vi "Retrieve Category SubPanel Information.vi"(8 "error in (no error)":errorcluster, 10 "ListBox Selection":i32, 11 "Configuration in":refnum<class "Configuration.lvclass">) -> (0 "error out":errorcluster, 1 "Help Text":string, 2 "VI Refnum":refnum<vi>, 3 "Configuration Out":refnum<class "Configuration.lvclass">)   [LabVIEW 2016, in "Configuration.lvlib" / "Configuration.lvclass"]
uses:
  <userlib>/Configuration Dialog Actor/Configuration.lvclass
  <userlib>/Configuration Dialog Actor/Configuration.lvclass/Configuration.ctl
  <userlib>/Configuration Dialog Actor/Methods/Data Retrieved by Lookup Table.ctl
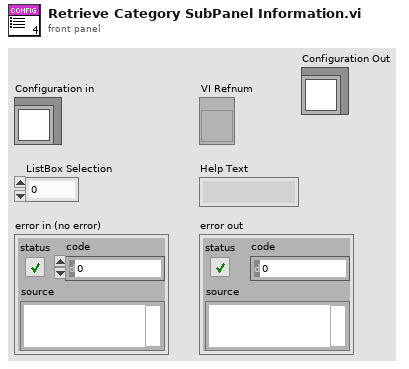
[diagram p1: front panel]
types:
  T1 = typedef "Configuration.lvlib/Configuration.lvclass/Data Retrieved by Lookup Table.ctl" = cluster{"VI Refnum":refnum<vi>, "Help Text":string}
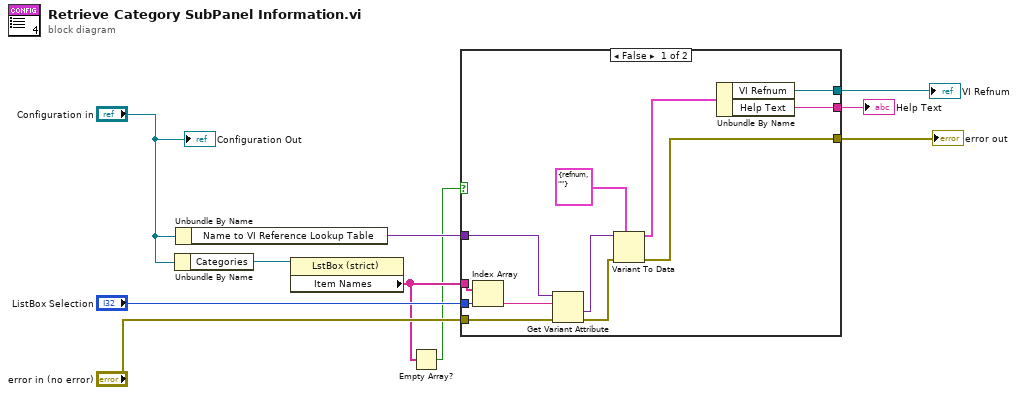
[diagram p0: block diagram]
diagram:
  n1 = Unbundle By Name("Configuration in") -> ("Categories"=w3:refnum<vi>)
  n2 = Unbundle By Name("Configuration in") -> ("Name to VI Reference Lookup Table"=w4:variant)
  n3 = property on="Property Node" class="LstBox (strict)"(reference=w3) -> ("Item Names"=w2:string[])  [unwired: 1 in, 2 out]
  n4 = Empty Array?(array=w2) -> (empty?=w1:bool)
  n5 = case shown="False" w1 {
    tunnel: [w22 _] -> w10
    tunnel: [w21 _] -> w9
    tunnel: "ListBox Selection" -> [w18 _]
    tunnel: [w16 w23] -> w6
    tunnel: "error in (no error)" -> [w15 w23]
    tunnel: w4 -> [w12 _]
    tunnel: w2 -> [w11 _]
    frame False {
      n6 = Index Array(array=w11, index=w18) -> (element=w13:string)
      n7 = Get Variant Attribute(Variant=w12, name=w13, error in=w15) -> (value=w14:variant, error out=w17:errorcluster)  [unwired: 1 in, 2 out]
      n8 = Variant To Data(error in=w17, type=T1 {"VI Refnum"=refnum, "Help Text"=""} ("output cluster"), Variant=w14) -> (data=w20:T1, error out=w16:errorcluster)
      n9 = Unbundle By Name(w20) -> ("VI Refnum"=w21:refnum<vi>, "Help Text"=w22:string)
    }
    frame True {
    }
  }
  "Help Text" <- w10
  "VI Refnum" <- w9
  "error out" <- w6
  "Configuration Out" <- "Configuration in"
